vi "Text to Timestamp(RFC3339).vi"(8 "error in (no error)":errorcluster, 9 "initial scan location":u32, 11 "Text Timestamp":string) -> (0 "error out":errorcluster, 1 "Offset Past Timestamp":u32, 2 "Local Time Offset (NaN if unspecified)":dbl, 3 "Time Stamp":timestamp format="%^<%H:%M:%S%6u\n%Y/%m/%d>T UTC")   [LabVIEW 2017, in "API String Arguments Support.lvlib"]
doc: "Supporting RFC3339, a subset of ISO8601, plus some other formats \nRFC3339--> https://tools.ietf.org/html/rfc3339 \n Examples:\n \"2020-06-25T08:50:15.123Z\"\n \"2020-06-25T09:50:15.123+01:00\"\n\nSQLite Time Functions --> https://www.sqlite.org/lang_datefunc.html\n Examples:\n \"2020-06-25 08:50:15\" --> datetime() function\n\nAlso accepts reduced formats omitting some of the separators, or replacing them with spaces:\n \"2020 06 25 085015Z\"\n\nTo support older versions of Windows Powershell (ConvertTo-Json commandlet), also supports milliseconds since the Unix Epoch, in /Date(nnn)/ format:\n \"/Date(1608992240123)/\""
uses:
  API String Arguments Support.lvlib
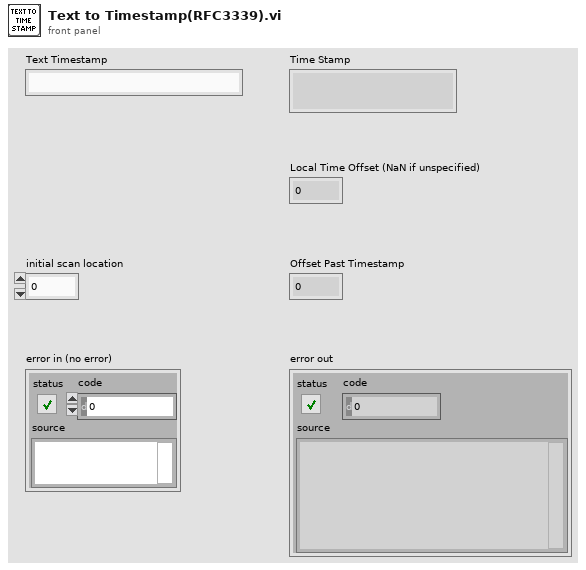
[diagram p1: front panel]
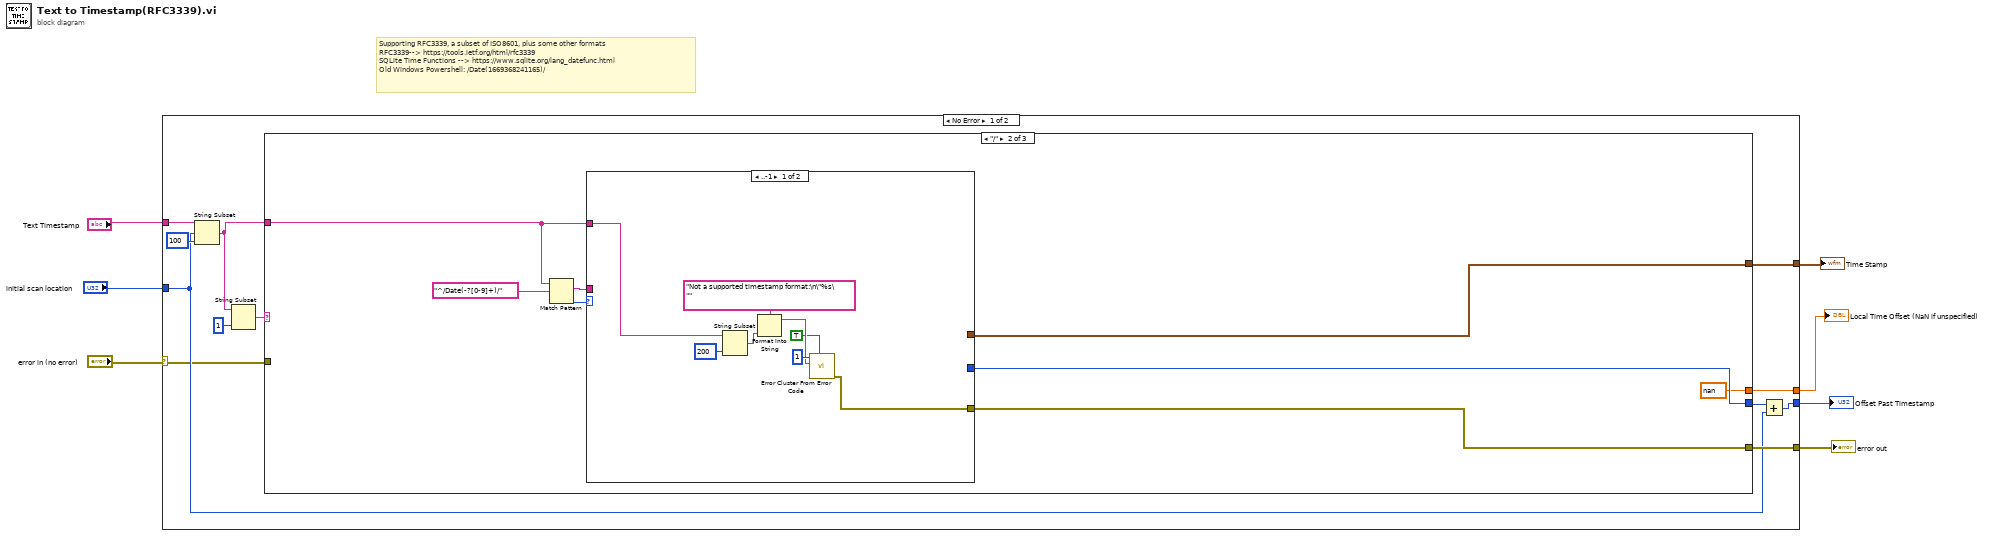
[diagram p0: block diagram]
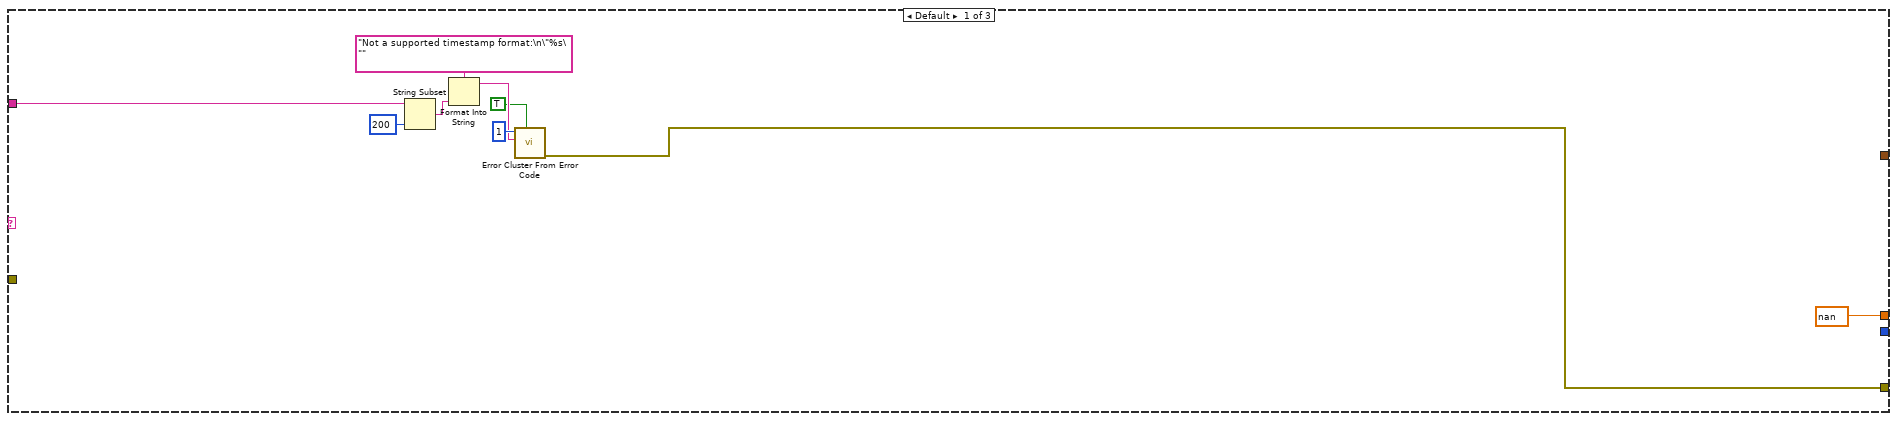
[diagram p2: hidden frame]
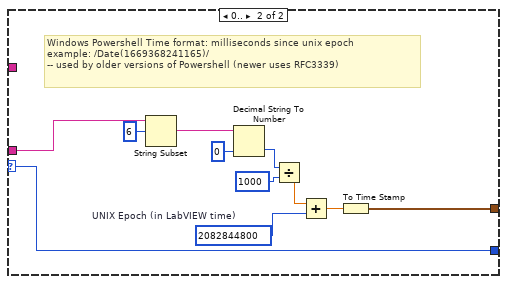
[diagram p3: hidden frame]
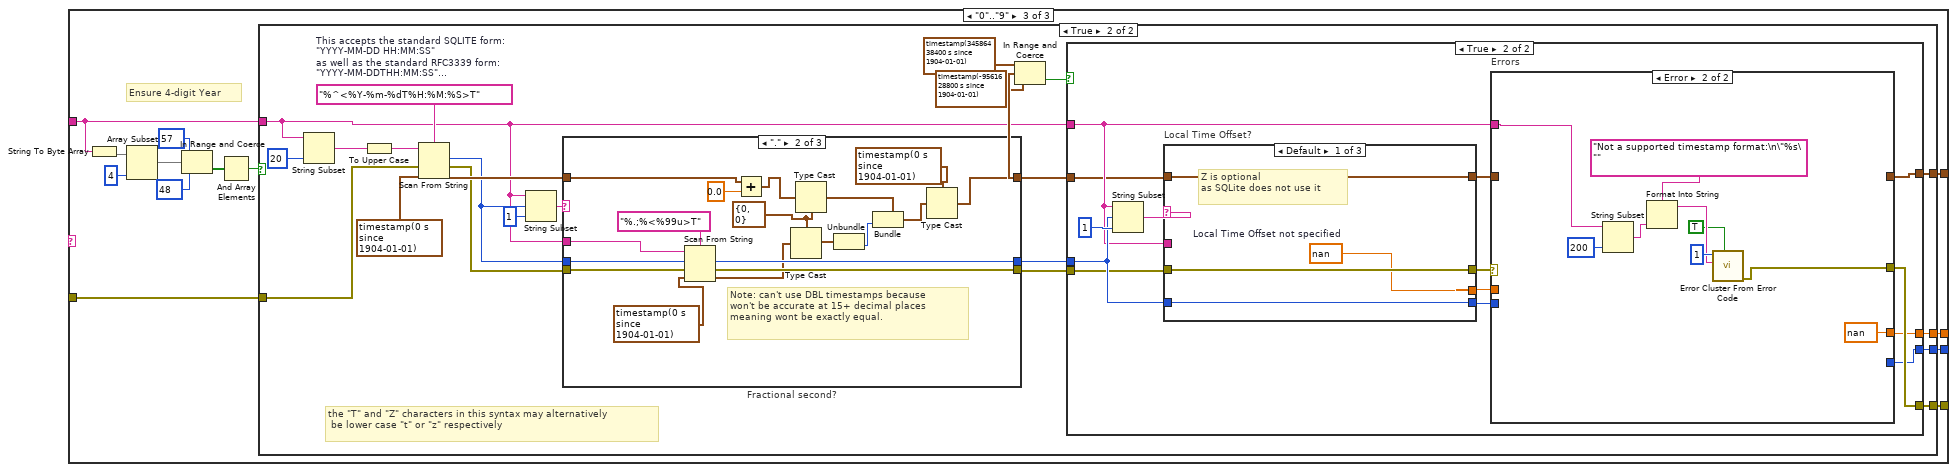
[diagram p4: hidden frame]
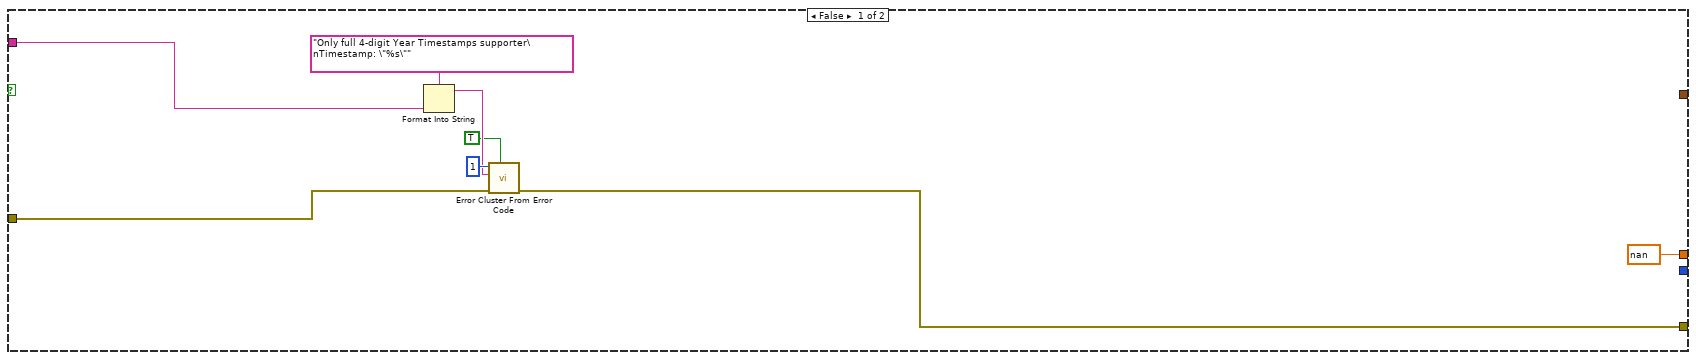
[diagram p5: hidden frame]
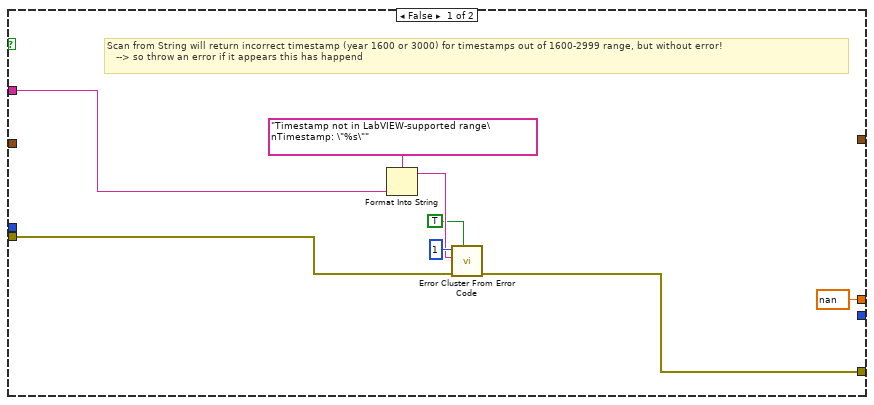
[diagram p6: hidden frame]
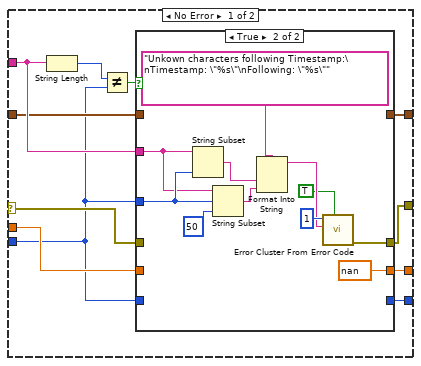
[diagram p7: hidden frame]
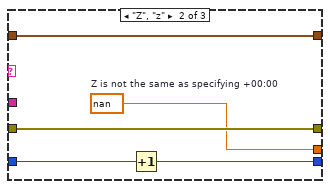
[diagram p9: hidden frame]
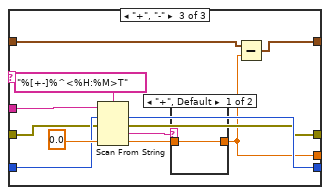
[diagram p10: hidden frame]
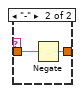
[diagram p11: hidden frame]
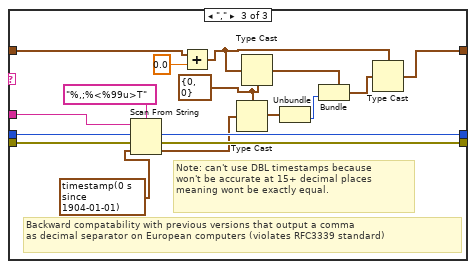
[diagram p13: hidden frame]
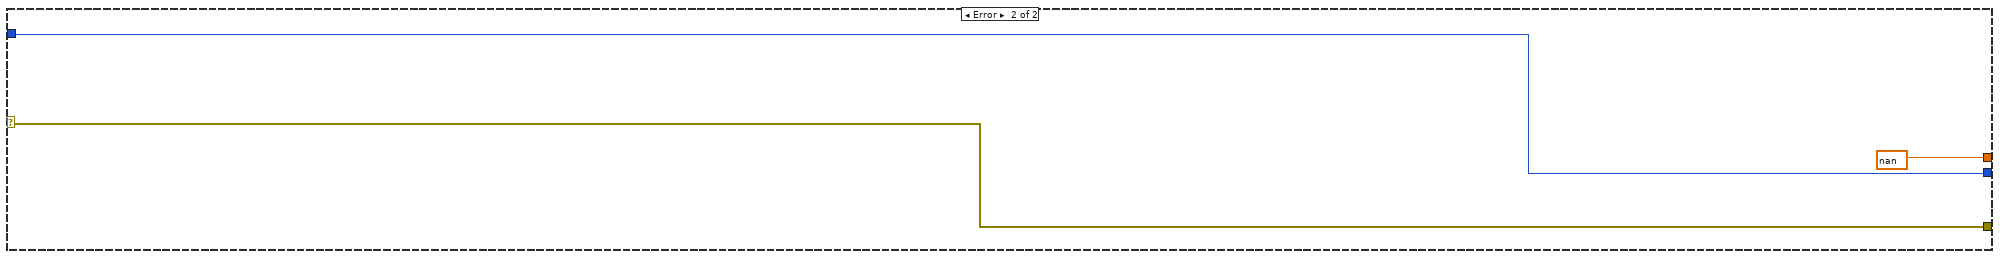
[diagram p14: hidden frame]
diagram:
  # "Supporting RFC3339, a subset of ISO8601, plus some other formats \nRFC3339--> https://tools.ietf.org/html/rfc3339\nSQLite Time Functions --> https://www.sqlite.org/lang_datefunc.html\nOld Windows Powershell: /Date(1669368241165)/"
  n1 = case shown="No Error" "error in (no error)" {
    selector: "error in (no error)" -> [w8 w218]
    tunnel: "Text Timestamp" -> [w14 _]
    tunnel: [w18 _] -> w6
    tunnel: [w9 w219] -> w1
    tunnel: [w19 w218] -> w5
    tunnel: [w17 nan] -> w3
    tunnel: "initial scan location" -> [w11 w219]
    frame No Error {
      n2 = String Subset(string=w14, offset (0)=w11, length (rest)=100 ("length (rest)")) -> (substring=w13:string)
      n3 = String Subset(string=w13, length (rest)=1 ("length (rest)")) -> (substring=w15:string)  [unwired: 1 in]
      n4 = case shown="\"/\"" w15 {
        tunnel: w8 -> [_ _ w68]
        tunnel: w13 -> [w28 w33 w63]
        tunnel: [w27 w32 w67] -> w19
        tunnel: [_ w31 w66] -> w18
        tunnel: [nan nan ("Z is not the same as specifying +00:00") w65] -> w17
        tunnel: [_ w30 w64] -> w10
        frame Default {
          n5 = String Subset(string=w28, length (rest)=200 ("length (rest)")) -> (substring=w23:string)  [unwired: 1 in]
          n6 = Format Into String(format string="Not a supported timestamp format:\n\"%s\"", w23) -> (resulting string=w21:string)  [unwired: 2 in, 1 out]
          n7 = call <vilib>:"Error Cluster From Error Code.vi"("show call chain? (False)"=TRUE, "error message (\"\")"=w21, "error code (0)"=1) -> ("error out"=w27:errorcluster)  [unwired: 6 in]
        }
        frame "/" {
          n8 = Match Pattern(string=w33, regular expression="^/Date(-?[0-9]+)/" ("format string")) -> (match substring=w35:string, offset past match=w34:i32)  [unwired: 1 in, 2 out]
          n9 = case shown="..-1" w34 {
            selector: w34 -> [_ w45]
            tunnel: w35 -> [_ w55]
            tunnel: [_ w46] -> w31
            tunnel: w33 -> [w44 _]
            tunnel: [w43 _] -> w32
            tunnel: [_ w45] -> w30
            frame ..-1 {
              n10 = String Subset(string=w44, length (rest)=200 ("length (rest)")) -> (substring=w40:string)  [unwired: 1 in]
              n11 = Format Into String(format string="Not a supported timestamp format:\n\"%s\"", w40) -> (resulting string=w38:string)  [unwired: 2 in, 1 out]
              n12 = call <vilib>:"Error Cluster From Error Code.vi"("show call chain? (False)"=TRUE, "error message (\"\")"=w38, "error code (0)"=1) -> ("error out"=w43:errorcluster)  [unwired: 6 in]
            }
            frame 0.. {
              w48 = i64 2082844800  # UNIX Epoch (in LabVIEW time)
              # "Windows Powershell Time format: milliseconds since unix epoch\nexample: /Date(1669368241165)/\n-- used by older versions of Powershell (newer uses RFC3339)"
              n13 = String Subset(string=w55, offset (0)=6) -> (substring=w53:string)  [unwired: 1 in]
              n14 = Decimal String To Number(string=w53, default (0L)=u64 0 ("default (0 I32)")) -> (number=w51:u64)  [unwired: 1 in, 1 out]
              n15 = Divide(x=w51, y=u64 1000) -> (x/y=w49:dbl)
              n16 = Add(x=w49, y=w48) -> (x+y=w47:dbl)
              n17 = To Time Stamp(1:w47) -> (0:w46:timestamp)
            }
          }
        }
        frame "0".."9" {
          # "Ensure 4-digit Year"
          n18 = String To Byte Array(string=w63) -> (unsigned byte array=w62:u8[])
          n19 = Array Subset(array=w62, length=4) -> (w60:u8[])  [unwired: 1 in]
          n20 = In Range and Coerce(upper limit=57, x=w60, lower limit=48) -> (In Range?=w57:bool[])  [unwired: 1 out]
          n21 = And Array Elements(Boolean array=w57) -> (logical AND=w56:bool)
          n22 = case shown="True" w56 {
            tunnel: w68 -> [w70 w92]
            tunnel: [w71 w89] -> w67
            tunnel: [_ w88] -> w66
            tunnel: [nan ("Z is not the same as specifying +00:00") w87] -> w65
            tunnel: [_ w86] -> w64
            tunnel: w63 -> [w69 w80]
            frame False {
              n23 = Format Into String(format string="Only full 4-digit Year Timestamps supporter\nTimestamp: \"%s\"", w69) -> (resulting string=w73:string)  [unwired: 2 in, 1 out]
              n24 = call <vilib>:"Error Cluster From Error Code.vi"("show call chain? (False)"=TRUE, "error in (no error)"=w70, "error message (\"\")"=w73, "error code (0)"=1) -> ("error out"=w71:errorcluster)  [unwired: 5 in]
            }
            frame True {
              w94 = "%^<%Y-%m-%dT%H:%M:%S>T"  # This accepts the standard SQLITE form: "YYYY-MM-DD HH:MM:SS"  as well as the standard RFC3339 form: "YYYY-MM-DDTHH:MM:SS" and ISO-8601 reduced forms that don't include some/all of the -, : or T: "YYYYMMDDHHMMSS"
              # "the \"T\" and \"Z\" characters in this syntax may alternatively\n be lower case \"t\" or \"z\" respectively"
              n25 = String Subset(string=w80, length (rest)=20 ("length (rest)")) -> (substring=w79:string)  [unwired: 1 in]
              n26 = To Upper Case(1:w79) -> (0:w81:string)
              n27 = Scan From String(format string=w94, input string=w81, error in=w92, default 1=timestamp(0 s since 1904-01-01)) -> (offset past scan=w77:u32, error out=w91:errorcluster, output 1=w95:timestamp)  [unwired: 1 in, 1 out]
              n28 = String Subset(string=w80, offset (0)=w77, length (rest)=1 ("length (rest)")) -> (substring=w96:string)
              n29 = case "Fractional second?" shown="\".\"" w96 {
                tunnel: w77 -> [w181 w197 w214]
                tunnel: w80 -> [_ w200 w217]
                tunnel: w95 -> [w182 w199 w216]
                tunnel: [w182 w198 w215] -> w85
                tunnel: [w181 w196 w213] -> w93
                tunnel: w91 -> [w180 w195 w212]
                tunnel: [w180 w194 w211] -> w90
                frame Default {
                }
                frame "." {
                  w189 = cluster{i64, u64} {0, 0}
                  # "Note: can't use DBL timestamps because\nwon't be accurate at 15+ decimal places\nmeaning wont be exactly equal."
                  n30 = Scan From String(format string="%.;%<%99u>T", input string=w200, initial scan location=w197, error in=w195, default 1=timestamp(0 s since 1904-01-01)) -> (offset past scan=w196:u32, error out=w194:errorcluster, output 1=w190:timestamp)  [unwired: 1 out]
                  n31 = Add(x=w199, y=0.0) -> (x+y=w184:timestamp)
                  n32 = Type Cast(type=w189, x=w190) -> (*(type *) &x=w187:cluster{i64, u64})
                  n33 = Type Cast(type=w189, x=w184) -> (*(type *) &x=w188:cluster{i64, u64})
                  n34 = Unbundle(w187) -> (w186:u64)  [unwired: 1 out]
                  n35 = Bundle(cluster=w188, w186) -> (w185:cluster{i64, u64})  [unwired: 1 in]
                  n36 = Type Cast(type=timestamp(0 s since 1904-01-01) ("x+y"), x=w185) -> (*(type *) &x=w198:timestamp)
                }
                frame "," {
                  w206 = cluster{i64, u64} {0, 0}
                  # "Backward compatability with previous versions that output a comma\nas decimal separator on European computers (violates RFC3339 standard)"
                  # "Note: can't use DBL timestamps because\nwon't be accurate at 15+ decimal places\nmeaning wont be exactly equal."
                  n37 = Scan From String(format string="%,;%<%99u>T", input string=w217, initial scan location=w214, error in=w212, default 1=timestamp(0 s since 1904-01-01)) -> (offset past scan=w213:u32, error out=w211:errorcluster, output 1=w207:timestamp)  [unwired: 1 out]
                  n38 = Add(x=w216, y=0.0) -> (x+y=w201:timestamp)
                  n39 = Type Cast(type=w206, x=w207) -> (*(type *) &x=w204:cluster{i64, u64})
                  n40 = Type Cast(type=w206, x=w201) -> (*(type *) &x=w205:cluster{i64, u64})
                  n41 = Unbundle(w204) -> (w203:u64)  [unwired: 1 out]
                  n42 = Bundle(cluster=w205, w203) -> (w202:cluster{i64, u64})  [unwired: 1 in]
                  n43 = Type Cast(type=w201, x=w202) -> (*(type *) &x=w215:timestamp)
                }
              }
              n44 = In Range and Coerce(upper limit=timestamp(34586438400 s since 1904-01-01), x=w85, lower limit=timestamp(-9561628800 s since 1904-01-01)) -> (In Range?=w82:bool)  [unwired: 1 out]
              n45 = case shown="True" w82 {
                tunnel: w93 -> [_ w118]
                tunnel: w90 -> [w101 w117]
                tunnel: [w100 w114] -> w89
                tunnel: [_ w112] -> w88
                tunnel: [nan ("Z is not the same as specifying +00:00") w110] -> w87
                tunnel: [_ w109] -> w86
                tunnel: w80 -> [w102 w108]
                tunnel: w85 -> [_ w107]
                frame False {
                  # "Scan from String will return incorrect timestamp (year 1600 or 3000) for timestamps out of 1600-2999 range, but without error!\n   --> so throw an error if it appears this has happend"
                  n46 = Format Into String(format string="Timestamp not in LabVIEW-supported range\nTimestamp: \"%s\"", w102) -> (resulting string=w104:string)  [unwired: 2 in, 1 out]
                  n47 = call <vilib>:"Error Cluster From Error Code.vi"("show call chain? (False)"=TRUE, "error in (no error)"=w101, "error message (\"\")"=w104, "error code (0)"=1) -> ("error out"=w100:errorcluster)  [unwired: 5 in]
                }
                frame True {
                  n48 = String Subset(string=w108, offset (0)=w118, length (rest)=1 ("length (rest)")) -> (substring=w119:string)
                  n49 = case "Local Time Offset?" shown="Default" w119 {
                    tunnel: w118 -> [w158 w163 w171]
                    tunnel: w108 -> [_ _ w175]
                    tunnel: w107 -> [w159 w164 w174]
                    tunnel: [w159 w164 w172] -> w113
                    tunnel: [w158 w162 w170] -> w116
                    tunnel: w117 -> [w157 w161 w169]
                    tunnel: [w157 w161 w168] -> w115
                    tunnel: [w156 w160 w166] -> w111
                    frame Default {
                      w156 = nan  # Local Time Offset not specified
                      # "Z is optional\nas SQLite does not use it"
                    }
                    frame "Z", "z" {
                      w160 = nan  # Z is not the same as specifying +00:00
                      n50 = Increment(x=w163) -> (x+1=w162:u32)
                    }
                    frame "+", "-" {
                      n51 = Scan From String(format string="%[+-]%^<%H:%M>T", input string=w175, initial scan location=w171, error in=w169, default 2=0.0) -> (offset past scan=w170:u32, error out=w168:errorcluster, output 1=w165:string, output 2=w167:dbl)  [unwired: 1 in, 1 out]
                      n52 = case shown="\"+\", Default" w165 {
                        tunnel: w167 -> [w177 w179]
                        tunnel: [w177 w178] -> w166
                        frame "+", Default {
                        }
                        frame "-" {
                          n53 = Negate(x=w179) -> (-x=w178:dbl)
                        }
                      }
                      n54 = Subtract(x=w174, y=w166) -> (x-y=w172:timestamp)
                    }
                  }
                  n55 = case "Errors" shown="Error" w115 {
                    selector: w115 -> [w127 _]
                    tunnel: w108 -> [w129 w155]
                    tunnel: w116 -> [w121 _]
                    tunnel: [w130 w154] -> w114
                    tunnel: w113 -> [w125 _]
                    tunnel: [w126 _] -> w112
                    tunnel: w111 -> [w124 _]
                    tunnel: [w123 nan] -> w110
                    tunnel: [w122 _] -> w109
                    frame No Error {
                      n56 = String Length(string=w129) -> (length=w131:i32)
                      n57 = Not Equal?(x=w131, y=w121) -> (x != y?=w128:bool)
                      n58 = case shown="True" w128 {
                        tunnel: [w135 w140] -> w130
                        tunnel: w121 -> [_ w139]
                        tunnel: w129 -> [_ w138]
                        tunnel: w127 -> [w135 _]
                        tunnel: [w134 _] -> w126
                        tunnel: w125 -> [w134 _]
                        tunnel: w124 -> [w133 _]
                        tunnel: [w133 nan] -> w123
                        tunnel: [w132 _] -> w122
                        tunnel: w121 -> [w132 _]
                        frame False {
                        }
                        frame True {
                          n59 = String Subset(string=w138, length (rest)=w139) -> (substring=w137:string)  [unwired: 1 in]
                          n60 = String Subset(string=w138, offset (0)=w139, length (rest)=50 ("length (rest)")) -> (substring=w144:string)
                          n61 = Format Into String(format string="Unkown characters following Timestamp:\nTimestamp: \"%s\"\nFollowing: \"%s\"", w137, w144) -> (resulting string=w142:string)  [unwired: 2 in, 1 out]
                          n62 = call <vilib>:"Error Cluster From Error Code.vi"("show call chain? (False)"=TRUE, "error message (\"\")"=w142, "error code (0)"=1) -> ("error out"=w140:errorcluster)  [unwired: 6 in]
                        }
                      }
                    }
                    frame Error {
                      n63 = String Subset(string=w155, length (rest)=200 ("length (rest)")) -> (substring=w150:string)  [unwired: 1 in]
                      n64 = Format Into String(format string="Not a supported timestamp format:\n\"%s\"", w150) -> (resulting string=w148:string)  [unwired: 2 in, 1 out]
                      n65 = call <vilib>:"Error Cluster From Error Code.vi"("show call chain? (False)"=TRUE, "error message (\"\")"=w148, "error code (0)"=1) -> ("error out"=w154:errorcluster)  [unwired: 6 in]
                    }
                  }
                }
              }
            }
          }
        }
      }
      n66 = Add(x=w10, y=w11) -> (x+y=w9:u32)
    }
    frame Error {
    }
  }
  "Time Stamp" <- w6
  "Offset Past Timestamp" <- w1
  "error out" <- w5
  "Local Time Offset (NaN if unspecified)" <- w3
